vi "DestroyPublicEvents.vi"(8 "error in (no error)":errorcluster, 11 "0MQ_Server":refnum<class "0MQ_Server.lvclass">) -> (0 "error out":errorcluster, 3 "0MQ_Server out":refnum<class "0MQ_Server.lvclass">)   [LabVIEW 2016, in "0MQ_Server.lvclass"]
doc: "JKI State Machine Objects (SMO) 1.0.0.7\nJKI - JKI\nCopyright (c) 2016, JKI"
uses:
  0MQ_Server.lvclass
  0MQ_Server.lvclass/0MQ_Server.ctl
  <vilib>/JKI/JKI SMO/SMO/SMO.lvclass
panel:
  # "For instructions on how to use the JKI State Machine Objects, examples and video tutorials, visit:\nhttp://jki.net/state-machine-objects/\n\nJKI State Machine Objects™\nhttp://jki.net/state-machine-objects/\nCopyright (C) 2005-2015, JKI <info@jki.net>\nALL RIGHTS RESERVED"
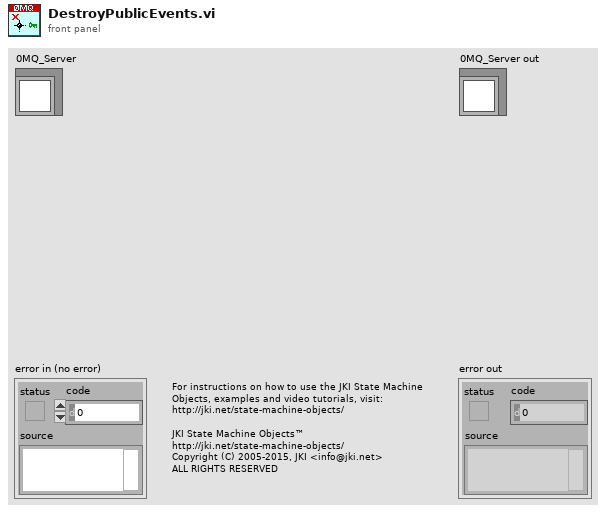
[diagram p1: front panel]
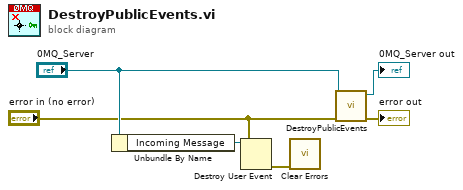
[diagram p0: block diagram]
diagram:
  n1 = Unbundle By Name("0MQ_Server") -> ("Incoming Message"=w3:refnum<user-event>)
  n2 = Destroy User Event(user event=w3, error in="error in (no error)") -> (error out=w1:errorcluster)
  n3 = call <vilib>:"Clear Errors.vi"("error in (no error)"=w1) -> ()  [unwired: 5 in, 2 out]
  n4 = call-parent "DestroyPublicEvents.vi"("error in (no error)"="error in (no error)", "SMO"="0MQ_Server") -> ("error out"=→"error out":errorcluster, "SMO out"=→"0MQ_Server out":refnum<class "0MQ_Server.lvclass">)  [unwired: 8 in]
